vi "38 Date Conversion (x64-2018).vi"(11 "Date In":string) -> (3 "Date Out":string)   [LabVIEW 2017]
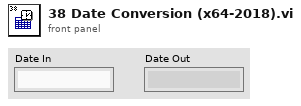
[diagram p1: front panel]
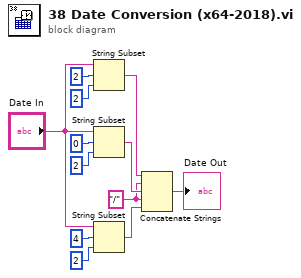
[diagram p0: block diagram]
diagram:
  w8 = "/"
  n1 = String Subset(string="Date In", offset (0)=2, length (rest)=2) -> (substring=w10:string)
  n2 = String Subset(string="Date In", offset (0)=0, length (rest)=2) -> (substring=w11:string)
  n3 = String Subset(string="Date In", offset (0)=4, length (rest)=2) -> (substring=w9:string)
  n4 = Concatenate Strings(w10, w8, w11, w8, w9) -> (→"Date Out":string)
